vi "Trigger.vi"(8 "error in (no error)":errorcluster, 10 "VNACluster In":T1={"Value"=0.0, "GUI Data Cluster"={"S11"=FALSE, "S21"=FALSE, "S12"=FALSE, "S22"=FALSE, "S11Meas"=enum."Log-magnitude (dB)", "S21Meas"=enum."Log-magnitude (dB)", "S12Meas"=enum."Log-magnitude (dB)", "S22Meas"=enum."Log-magnitude (dB)", "S11Param"=enum."S11", "S21Param"=enum."S21", "S12Param"=enum."S12", "S22Param"=enum."S22"}, "Timing"={"Last Operation"=0.0, "Stop @ T/B"=FALSE, "Last Temp"=0.0, "Last Mag"=0.0, "Ramp Param"={"End T (K)"=0.0, "Delta T (K)"=0.0, "End B (T)"=0.0, "Delta B (T)"=0.0}, "LastOp?"=FALSE, "FirstOp?"=FALSE}, "Measurements"=[], "Hardware"={"VNA TCP Con"=refnum, "VNA TCP Port"=5025, "Global T VAR"="", "Global B VAR"=""}, "Operation"={"Operation Mode"=enum."Logging", "Log Folder"=path "", "Measure Mode"=enum."Deltat"}}) -> (0 "error out":errorcluster, 1 "TriggerTime":timestamp, 2 "VNACluster Out":T1={"Value"=0.0, "GUI Data Cluster"={"S11"=FALSE, "S21"=FALSE, "S12"=FALSE, "S22"=FALSE, "S11Meas"=enum."Log-magnitude (dB)", "S21Meas"=enum."Log-magnitude (dB)", "S12Meas"=enum."Log-magnitude (dB)", "S22Meas"=enum."Log-magnitude (dB)", "S11Param"=enum."S11", "S21Param"=enum."S21", "S12Param"=enum."S12", "S22Param"=enum."S22"}, "Timing"={"Last Operation"=0.0, "Stop @ T/B"=FALSE, "Last Temp"=0.0, "Last Mag"=0.0, "Ramp Param"={"End T (K)"=0.0, "Delta T (K)"=0.0, "End B (T)"=0.0, "Delta B (T)"=0.0}, "LastOp?"=FALSE, "FirstOp?"=FALSE}, "Measurements"=[], "Hardware"={"VNA TCP Con"=refnum, "VNA TCP Port"=5025, "Global T VAR"="", "Global B VAR"=""}, "Operation"={"Operation Mode"=enum."Logging", "Log Folder"=path "", "Measure Mode"=enum."Deltat"}})   [LabVIEW 2021]
uses:
  Sources/Data_Cluster.ctl
  Sources/Measurement_Cluster.ctl
  Sources/Mode_Enum.ctl
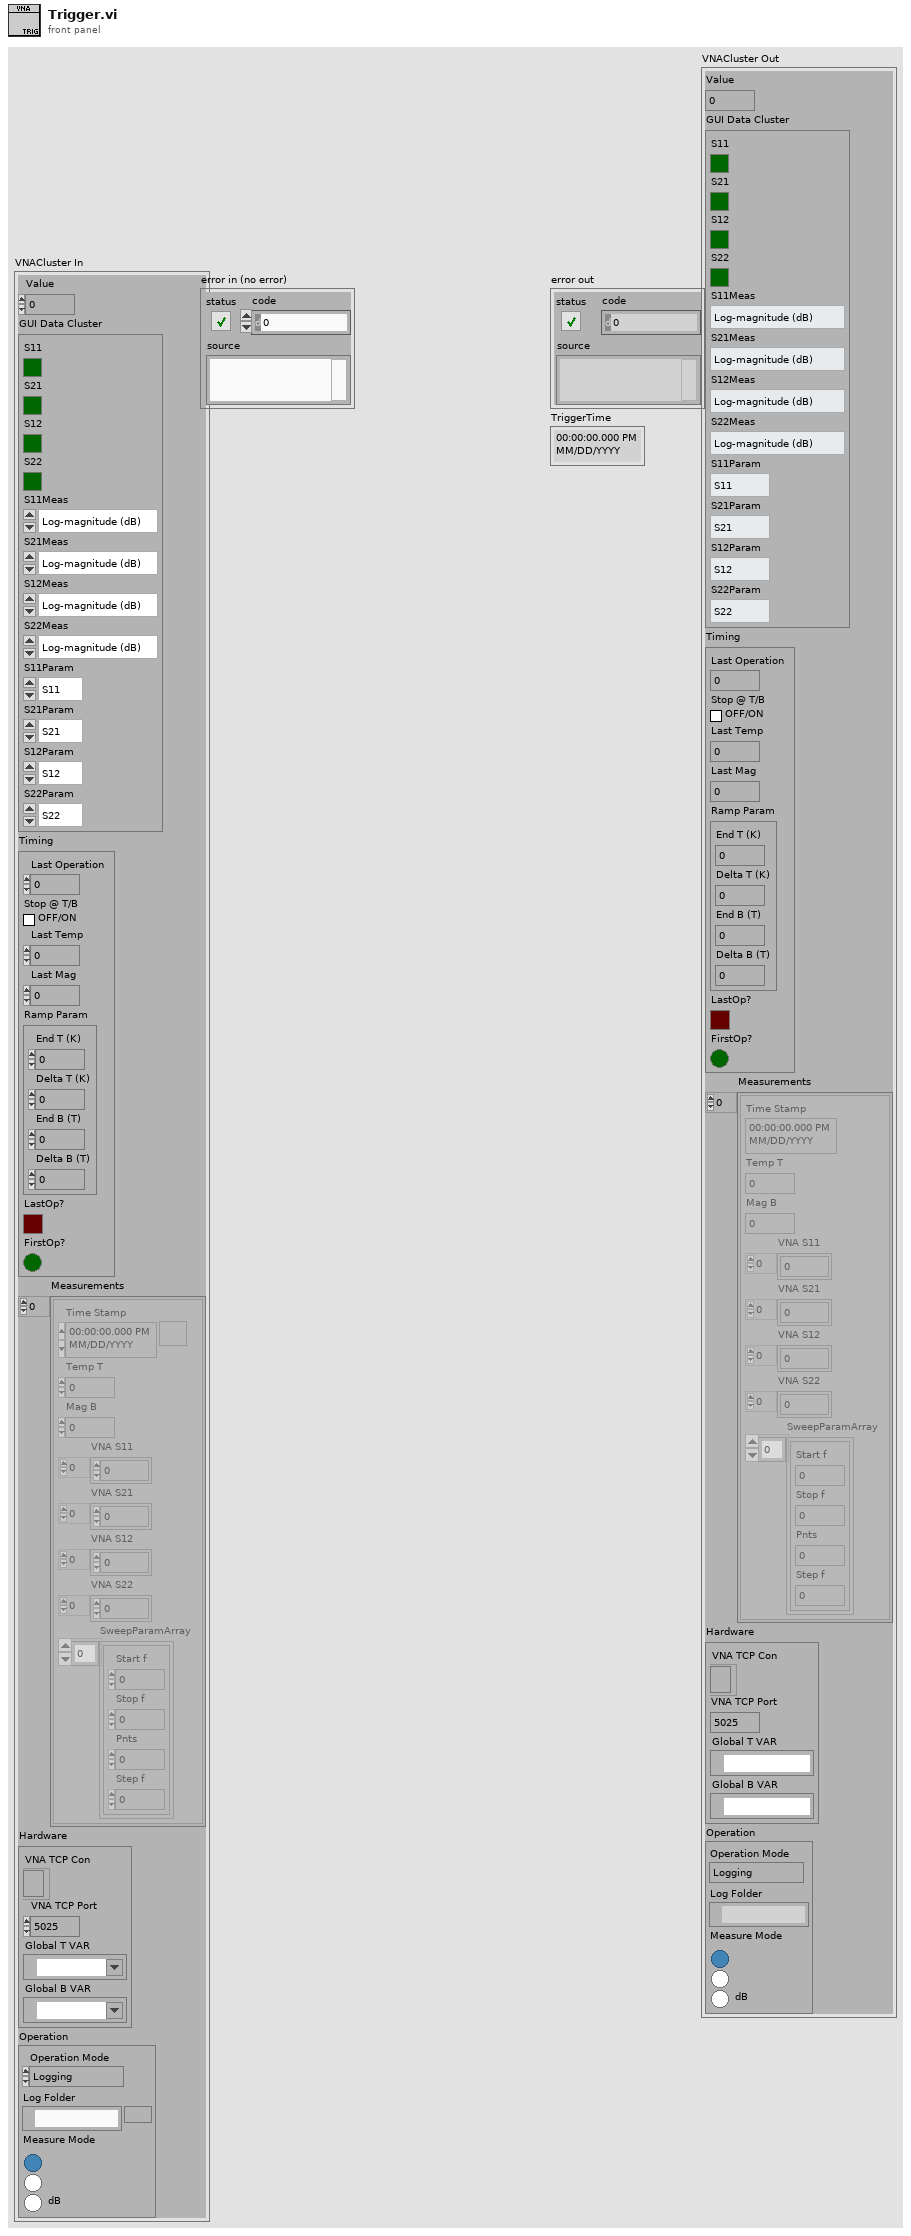
[diagram p1: front panel]
types:
  T1 = typedef "Data_Cluster.ctl" = cluster{"Value":dbl, "GUI Data Cluster":cluster{"S11":bool, "S21":bool, "S12":bool, "S22":bool, "S11Meas":enum16{"Log-magnitude (dB)", "Linear magnitude", "Phase (deg)", "Time Domain", "Real", "Imaginary", "Group Delay", "Polarlinear"}, "S21Meas":enum16{"Log-magnitude (dB)", "Linear magnitude", "Phase (deg)", "Time Domain", "Real", "Imaginary", "Group Delay", "Polarlinear"}, "S12Meas":enum16{"Log-magnitude (dB)", "Linear magnitude", "Phase (deg)", "Time Domain", "Real", "Imaginary", "Group Delay", "Polarlinear"}, "S22Meas":enum16{"Log-magnitude (dB)", "Linear magnitude", "Phase (deg)", "Time Domain", "Real", "Imaginary", "Group Delay", "Polarlinear"}, "S11Param":enum16{"S11", "S21", "S12", "S22"}, "S21Param":enum16{"S11", "S21", "S12", "S22"}, "S12Param":enum16{"S11", "S21", "S12", "S22"}, "S22Param":enum16{"S11", "S21", "S12", "S22"}}, "Timing":cluster{"Last Operation":dbl, "Stop @ T/B":bool, "Last Temp":dbl, "Last Mag":dbl, "Ramp Param":cluster{"End T (K)":dbl, "Delta T (K)":dbl, "End B (T)":dbl, "Delta B (T)":dbl}, "LastOp?":bool, "FirstOp?":bool}, "Measurements":T2[], "Hardware":cluster{"VNA TCP Con":refnum<k5>, "VNA TCP Port":i32, "Global T VAR":refnum<k21>, "Global B VAR":refnum<k21>}, "Operation":cluster{"Operation Mode":T3, "Log Folder":path, "Measure Mode":enum32{"Deltat", "DeltaT", "dB"}}}
  T2 = typedef "Measurement_Cluster.ctl" = cluster{"Time Stamp":timestamp, "Temp T":dbl, "Mag B":dbl, "VNA S11":dbl[], "VNA S21":dbl[], "VNA S12":dbl[], "VNA S22":dbl[], "SweepParamArray":cluster{"Start f":dbl, "Stop f":dbl, "Pnts":i32, "Step f":dbl}[]}
  T3 = typedef "Mode_Enum.ctl" = enum16{"Logging", "Idle-Off", "Idle"}
  T4 = enum16{"Standard", "Buffered", "CRLF", "Immediate"}
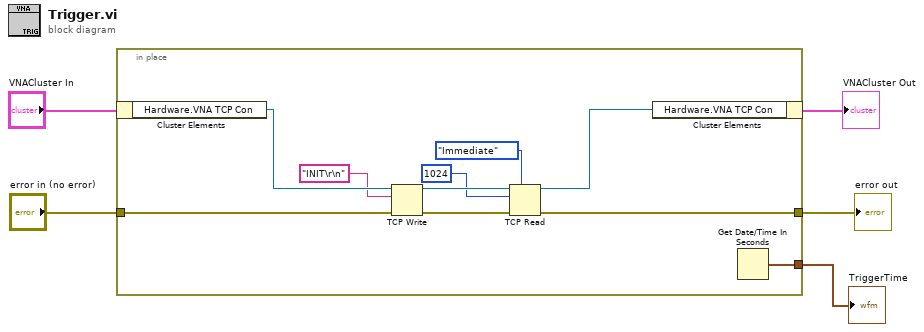
[diagram p0: block diagram]
diagram:
  n1 = in-place {
    in-place-border: "error in (no error)" -> [w15]
    in-place-border: [w7] -> w2
    in-place-border: [w6] -> w1
    n2 = in-place-cluster #1("VNACluster In") -> ("Hardware.VNA TCP Con"=w14:refnum<k5>)
    n3 = TCP Write(connection ID=w14, data in="INIT\r\n", error in (no error)=w15) -> (connection ID out=w12:refnum<k5>, error out=w13:errorcluster)  [unwired: 1 in, 1 out]
    n4 = TCP Read(connection ID=w12, bytes to read=1024, error in (no error)=w13, 7:T4."Immediate" ("mode (standard)")) -> (connection ID out=w8:refnum<k5>, error out=w7:errorcluster)  [unwired: 1 in, 1 out]
    n5 = in-place-cluster #1("Hardware.VNA TCP Con"=w8) -> (→"VNACluster Out":T1)
    n6 = Get Date/Time In Seconds() -> (seconds since 1Jan1904=w6:timestamp)
  }
  "error out" <- w2
  "TriggerTime" <- w1
